vi "Write Combination.vi"(8 "error in (no error)":errorcluster, 10 "Combination":T1[](array[typedef]), 11 "Cheat in":refnum<class "Cheat.lvclass">) -> (0 "error out":errorcluster, 3 "Cheat out":refnum<class "Cheat.lvclass">)   [LabVIEW 2019, in "RT_Game.lvlib" / "Cheat.lvclass"]
uses:
  Cheat.lvclass
  CheatControl.ctl
  Cheat.lvclass/Cheat.ctl
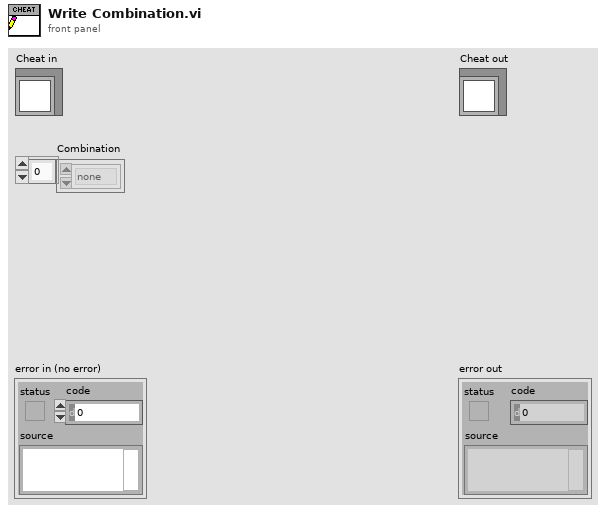
[diagram p1: front panel]
types:
  T1 = typedef "RT_Game.lvlib/Cheat.lvclass/CheatControl.ctl" = enum16{"none", "left1", "left2", "right1", "right2", "leftStick", "rightStick"}
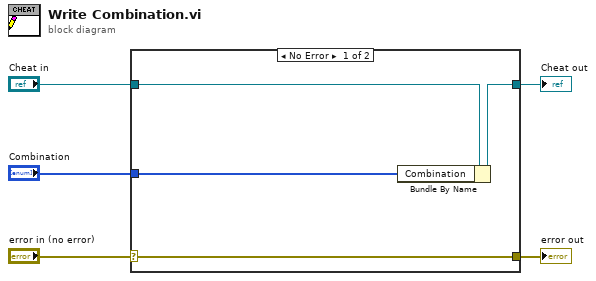
[diagram p0: block diagram]
diagram:
  n1 = case shown="No Error" "error in (no error)" {
    selector: "error in (no error)" -> [w9 w10]
    tunnel: [w9 w10] -> w4
    tunnel: [w7 w11] -> w2
    tunnel: "Cheat in" -> [w8 w11]
    tunnel: "Combination" -> [w6 _]
    frame No Error {
      n2 = Bundle By Name(cluster=w8, "Combination"=w6) -> (w7:refnum<class "Cheat.lvclass">)
    }
    frame Error {
    }
  }
  "error out" <- w4
  "Cheat out" <- w2
